vi "XY Graph Append Point to Plot.vi"(4 "Create Plot? (T)":bool=TRUE, 6 "Plot ID (-1: last)":i32=-1, 7 "overwrite point at x? (T)":bool=TRUE, 8 "error in (no error)":errorcluster, 9 "y":dbl, 10 "x":dbl, 11 "XYGraph in":refnum<vi>) -> (0 "error out":errorcluster, 1 "# Plots":i32, 2 "Actual Plot ID":i32, 3 "Plot Created?":bool)   [LabVIEW 2021, in "XY Graph Add-Ons.lvlib"]
uses:
  XY Graph Add-Ons.lvlib
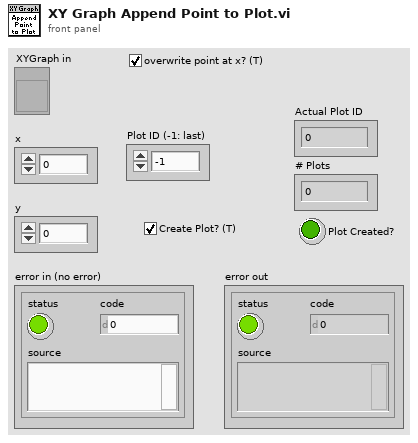
[diagram p1: front panel]
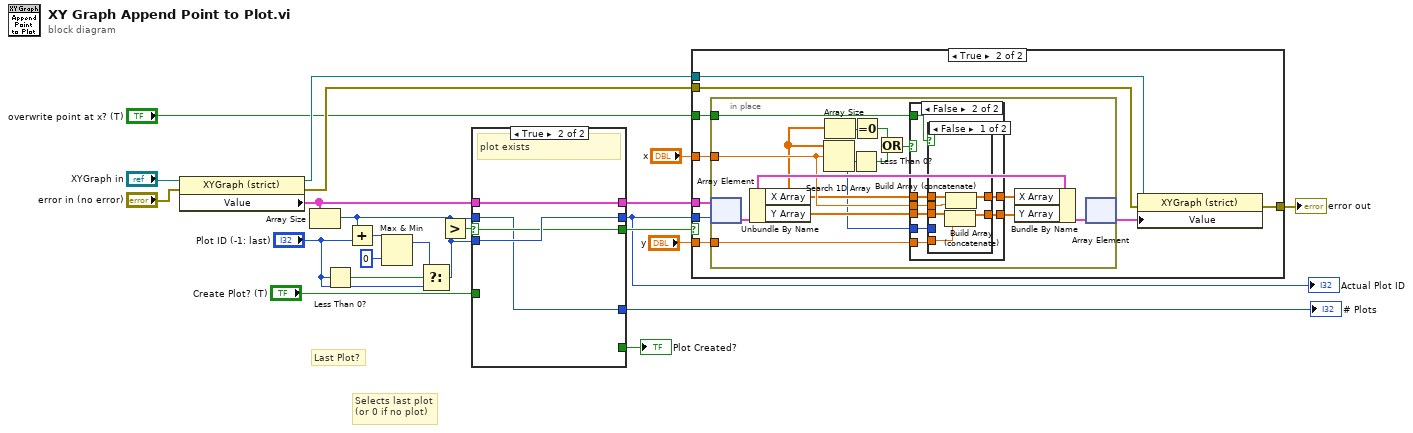
[diagram p0: block diagram]
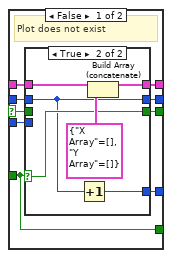
[diagram p2: hidden frame]
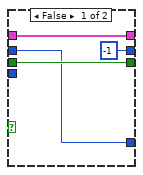
[diagram p3: hidden frame]
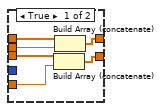
[diagram p5: hidden frame]
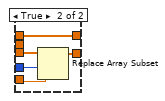
[diagram p6: hidden frame]
diagram:
  # "Selects last plot\n(or 0 if no plot)"
  # "Last Plot?"
  n1 = property class="XYGraph (strict)"(reference="XYGraph in", error in="error in (no error)") -> (reference out=w18:refnum<vi>, error out=w17:errorcluster, "Value"=w15:cluster{"X Array":dbl[], "Y Array":dbl[]}[])
  n2 = Array Size(array=w15) -> (size(s)=w5:i32)
  n3 = Less Than 0?(x="Plot ID (-1: last)") -> (x < 0?=w9:bool)
  n4 = Add(x=w5, y="Plot ID (-1: last)") -> (x+y=w3:i32)
  n5 = Max & Min(x=w3, y=0) -> (max(x,y)=w7:i32)  [unwired: 1 out]
  n6 = Select(t=w7, s=w9, f="Plot ID (-1: last)") -> (s? t:f=w6:i32)
  n7 = Greater?(x=w5, y=w6) -> (0:w16:bool)
  n8 = case shown="True" w16 {
    selector: w16 -> [w27 w44]
    tunnel: w15 -> [w29 w46]
    tunnel: [w28 w46] -> w14
    tunnel: w5 -> [w31 w43]
    tunnel: [w30 w45] -> w10
    tunnel: "Create Plot? (T)" -> [w24 _]
    tunnel: w6 -> [w32 w45]
    tunnel: [w26 w44] -> w12
    tunnel: [w25 w43] -> w11
    tunnel: [w24 _] -> w2
    frame False {
      # "Plot does not exist"
      n9 = case shown="True" w24 {
        selector: w24 -> [_ w39]
        tunnel: w32 -> [_ _]
        tunnel: w31 -> [w33 w38]
        tunnel: [-1 w38] -> w30
        tunnel: w29 -> [w36 w42]
        tunnel: [w36 w41] -> w28
        tunnel: w27 -> [w34 _]
        tunnel: [w34 w39] -> w26
        tunnel: [w33 w37] -> w25
        frame False {
        }
        frame True {
          n10 = Increment(x=w38) -> (x+1=w37:i32)
          n11 = Build Array (concatenate)(w42, cluster{"X Array":dbl[], "Y Array":dbl[]} {"X Array"=[], "Y Array"=[]} ("Value")) -> (w41:cluster{"X Array":dbl[], "Y Array":dbl[]}[])
        }
      }
    }
    frame True {
      # "plot exists"
    }
  }
  "# Plots" <- w11
  "Actual Plot ID" <- w10
  "Plot Created?" <- w2
  n12 = case shown="True" w12 {
    tunnel: [w47 w56] -> w23
    tunnel: "y" -> [_ w55]
    tunnel: "x" -> [_ w54]
    tunnel: w14 -> [_ w52]
    tunnel: w18 -> [_ w51]
    tunnel: w17 -> [w47 w50]
    tunnel: w10 -> [_ w49]
    tunnel: "overwrite point at x? (T)" -> [_ w48]
    frame False {
    }
    frame True {
      n13 = in-place {
        in-place-border: w54 -> [w64]
        in-place-border: w55 -> [w69]
        in-place-border: w48 -> [w57]
        n14 = in-place-array #1(w52, w49) -> (w68:cluster{"X Array":dbl[], "Y Array":dbl[]})
        n15 = Unbundle By Name(w68) -> ("X Array"=w63:dbl[], "Y Array"=w70:dbl[])
        n16 = Search 1D Array(1D array=w63, element=w64) -> (index of element=w58:i32)  [unwired: 1 in]
        n17 = Array Size(array=w63) -> (size(s)=w62:i32)
        n18 = Less Than 0?(x=w58) -> (x < 0?=w60:bool)
        n19 = Equal To 0?(x=w62) -> (x = 0?=w61:bool)
        n20 = Or(x=w61, y=w60) -> (x .or. y?=w59:bool)
        n21 = case shown="False" w59 {
          tunnel: w70 -> [w76 w84]
          tunnel: w69 -> [w75 w83]
          tunnel: [w74 w78] -> w67
          tunnel: [w73 w82] -> w66
          tunnel: w63 -> [w72 w79]
          tunnel: w64 -> [w71 w77]
          tunnel: w58 -> [_ w81]
          tunnel: w57 -> [_ w80]
          frame True {
            n22 = Build Array (concatenate)(w76, w75) -> (w73:dbl[])
            n23 = Build Array (concatenate)(w72, w71) -> (w74:dbl[])
          }
          frame False {
            n24 = case shown="False" w80 {
              tunnel: w84 -> [w87 w95]
              tunnel: w83 -> [w86 w94]
              tunnel: [w85 w93] -> w82
              tunnel: w81 -> [_ w92]
              tunnel: w79 -> [w90 w91]
              tunnel: [w88 w91] -> w78
              tunnel: w77 -> [w89 _]
              frame False {
                n25 = Build Array (concatenate)(w87, w86) -> (w85:dbl[])
                n26 = Build Array (concatenate)(w90, w89) -> (w88:dbl[])
              }
              frame True {
                n27 = Replace Array Subset(array=w95, new element=w94, index=w92) -> (w93:dbl[])
              }
            }
          }
        }
        n28 = Bundle By Name(cluster=w68, "X Array"=w67, "Y Array"=w66) -> (w65:cluster{"X Array":dbl[], "Y Array":dbl[]})
        n29 = in-place-array #1(w65) -> (w53:cluster{"X Array":dbl[], "Y Array":dbl[]}[])  [unwired: 1 out]
      }
      n30 = property class="XYGraph (strict)"(reference=w51, error in=w50, "Value"=w53) -> (error out=w56:errorcluster)  [unwired: 1 out]
    }
  }
  "error out" <- w23
